vi "5492_AutonomousStraightTuning.vi"(10 "Straight Type":string="Numeric") -> (2 "Done":bool)   [LabVIEW 2017]
uses:
  5492_WPI_RobotDriveMotorSelectorEnum.ctl
  <vilib>/Rock Robotics/WPI/ThirdParty/Cross The Road Electronics/Phoenix-LabVIEW/Motor Controller/Controls/CTRE_Phoenix_MotorControl_ControlMode.ctl
  <vilib>/Rock Robotics/WPI/Utilities/WPI_GetSetVariantRefNum.vi
  <vilib>/Rock Robotics/Network Tables/NT Read Number.vi
  <vilib>/Rock Robotics/WPI/RobotDrive/WPI_RobotDriveSafetyCheck.vi
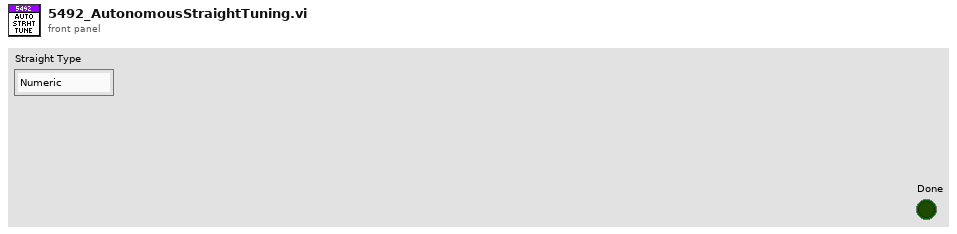
[diagram p1: front panel]
types:
  T1 = typedef "5492_WPI_RobotDriveMotorSelectorEnum.ctl" = enum16{"Front left motor", "Front right motor"}
  T2 = typedef "WPI_RobotDriveDevRef.ctl" = cluster{"DevStatus":errorcluster, "Motors[]":T3[], "Square Inputs":bool, "Max Output":dbl}
  T3 = typedef "WPI_MotorControlDeviceRef.ctl" = cluster{"DeviceStatus":errorcluster, "Type":T4, "PWM":cluster{"PWM Channel":T5, "DeadBand":T6}, "CAN":cluster{"Device Number":u8, "SetOutput VI Ref":variant, "GetOutput VI Ref":variant, "Enable VI Ref":variant, "Disable VI Ref":variant, "Data":variant}, "Invert":bool, "DIO PWM":cluster{"PWM \"Enable\" Channel":T5, "DIOChannel":T7, "PWM Rate":dbl}}
  T4 = typedef "WPI_MotorControlType.ctl" = enum16{"PWM", "CAN", "DIO PWM"}
  T5 = typedef "FPGA_DIOPWMChannel.ctl" = enum8{"PWM 0", "PWM 1", "PWM 2", "PWM 3", "PWM 4", "PWM 5", "PWM 6", "PWM 7", "PWM 8", "PWM 9", "PWM MXP 0", "PWM MXP 1", "PWM MXP 2", "PWM MXP 3", "PWM MXP 4", "PWM MXP 5", "PWM MXP 6", "PWM MXP 7", "PWM MXP 8", "PWM MXP 9", "Invalid"}
  T6 = typedef "WPI_PWMDeadband.ctl" = cluster{"Name":string, "maxPositivePwm":i32, "minPositivePwm":i32, "centerPwm":i32, "maxNegativePwm":i32, "minNegativePwm":i32, "angularRange":u16}
  T7 = typedef "FPGA_DIOChannel.ctl" = enum8{"DIO 0", "DIO 1", "DIO 2", "DIO 3", "DIO 4", "DIO 5", "DIO 6", "DIO 7", "DIO 8", "DIO 9", "DIO MXP 0", "DIO MXP 1", "DIO MXP 2", "DIO MXP 3", "DIO MXP 4", "DIO MXP 5", "DIO MXP 6", "DIO MXP 7", "DIO MXP 8", "DIO MXP 9", "DIO MXP 10", "DIO MXP 11", "DIO MXP 12", "DIO MXP 13", "DIO MXP 14", "DIO MXP 15", "SPI Port CS1", "SPI Port CS2", "SPI Port CS3", "SPI Port MISO", "SPI Port MOSI", "Invalid"}
  T8 = typedef "CTRE_Phoenix_MotorControl_ControlMode.ctl" = u16
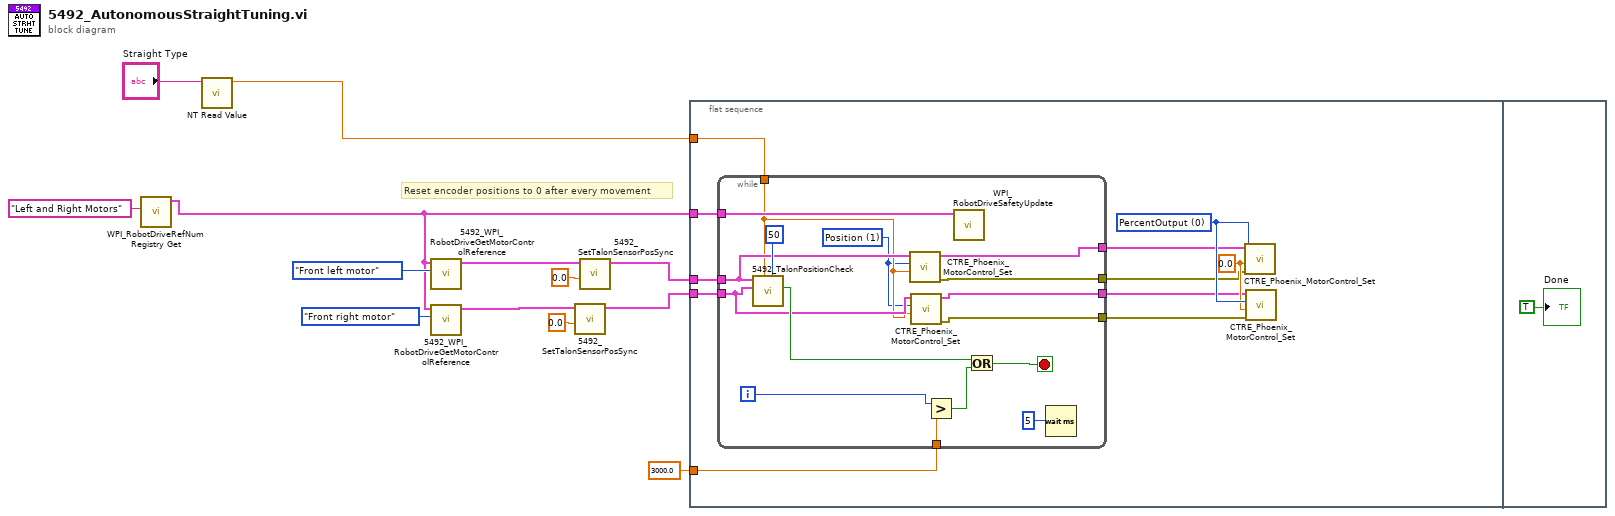
[diagram p0: block diagram]
diagram:
  # "Reset encoder positions to 0 after every movement"
  n1 = call <vilib>:"WPI_RobotDriveRefNum Registry Get.vi"("refnum name"="Left and Right Motors") -> ("RobotDriveDevRef"=w4:T2)  [unwired: 9 in, 1 out]
  n2 = call-poly <vilib>:"NT Read Value.vi"("Name"="Straight Type") -> ("Numeric"=w3:dbl)  [unwired: 9 in, 1 out]
  n3 = call "5492_WPI_RobotDriveGetMotorControlReference.vi"("MotorIndex"=5492_WPI_RobotDriveMotorSelectorEnum."Front left motor", "RobotDriveDevRef"=w4) -> ("MotorControlDeviceRef"=w10:T3)  [unwired: 9 out]
  n4 = call "5492_WPI_RobotDriveGetMotorControlReference.vi"("MotorIndex"=5492_WPI_RobotDriveMotorSelectorEnum."Front right motor", "RobotDriveDevRef"=w4) -> ("MotorControlDeviceRef"=w8:T3)  [unwired: 9 out]
  n5 = call "5492_SetTalonSensorPosSync.vi"("Pos"=0.0 ("New Sensor Position"), "CAN Talon SRX Ref In"=w8) -> ("CAN Talon SRX Ref Out"=w7:T3)  [unwired: 8 in, 1 out]
  n6 = call "5492_SetTalonSensorPosSync.vi"("Pos"=0.0 ("New Sensor Position"), "CAN Talon SRX Ref In"=w10) -> ("CAN Talon SRX Ref Out"=w6:T3)  [unwired: 8 in, 1 out]
  n7 = flat-sequence {
    tunnel: w7 -> [w24]
    tunnel: w6 -> [w23]
    tunnel: 3000.0 ("Numeric") -> [w22]
    tunnel: w3 -> [w21]
    tunnel: w4 -> [w20]
    frame #0 {
      w19 = T8 0 items=["PercentOutput"=0, "Position"=1, "Velocity"=2, "Current"=3, "Follower"=5, "MotionProfile"=6, "MotionMagic"=7, "MotionMagicArc"=8, "MotionProfileArc"=10, "Disabled"=15] ("Control Mode")
      w18 = 0.0 ("Output")
      n8 = while {
        tunnel: w24 -> [w31]
        tunnel: w23 -> [w32]
        tunnel: w22 -> [w36]
        tunnel: w21 -> [w30]
        tunnel: w20 -> [w33]
        tunnel: [w28] -> w17
        tunnel: [w27] -> w16
        tunnel: [w26] -> w15
        tunnel: [w25] -> w14
        i -> [w37]
        stop <- w40 stop-if-true
        w29 = T8 1 items=["PercentOutput"=0, "Position"=1, "Velocity"=2, "Current"=3, "Follower"=5, "MotionProfile"=6, "MotionMagic"=7, "MotionMagicArc"=8, "MotionProfileArc"=10, "Disabled"=15] ("Control Mode")
        n9 = call "5492_TalonPositionCheck.vi"("Margin of Error"=50, "Position Goal"=w30, "CAN Talon SRX Ref Right"=w31, "CAN Talon SRX Ref Left"=w32) -> ("Goal Achieved"=w39:bool)  [unwired: 7 in]
        n10 = call <vilib>:"CTRE_Phoenix_MotorControl_Set.vi"("Output"=w30, "Control Mode"=w29, "PhoenixMotorControlDevRef"=w32) -> ("error out"=w26:errorcluster, "PhoenixMotorControlDevRef"=w28:T3)  [unwired: 7 in]
        n11 = call <vilib>:"CTRE_Phoenix_MotorControl_Set.vi"("Output"=w30, "Control Mode"=w29, "PhoenixMotorControlDevRef"=w31) -> ("error out"=w25:errorcluster, "PhoenixMotorControlDevRef"=w27:T3)  [unwired: 7 in]
        n12 = Greater?(x=w37, y=w36) -> (0:w38:bool)
        n13 = call <vilib>:"WPI_RobotDriveSafetyUpdate.vi"("RobotDriveDevRef"=w33) -> ()  [unwired: 1 in, 10 out]
        n14 = Or(x=w39, y=w38) -> (x .or. y?=w40:bool)
        n15 = Wait (ms)(milliseconds to wait=u32 5) -> ()  [unwired: 1 out]
      }
      n16 = call <vilib>:"CTRE_Phoenix_MotorControl_Set.vi"("error in (no error)"=w15, "Output"=w18, "Control Mode"=w19, "PhoenixMotorControlDevRef"=w17) -> ()  [unwired: 6 in, 2 out]
      n17 = call <vilib>:"CTRE_Phoenix_MotorControl_Set.vi"("error in (no error)"=w14, "Output"=w18, "Control Mode"=w19, "PhoenixMotorControlDevRef"=w16) -> ()  [unwired: 6 in, 2 out]
    }
    frame #1 {
      "Done" <- TRUE ("Done")
    }
  }
